vi "运行模式.vi"() -> (3 "单机运行":bool)   [LabVIEW 2014]
panel:
  in  "单机运行":bool
  in  "联机运行":bool
  # "请选择一种运行方式"
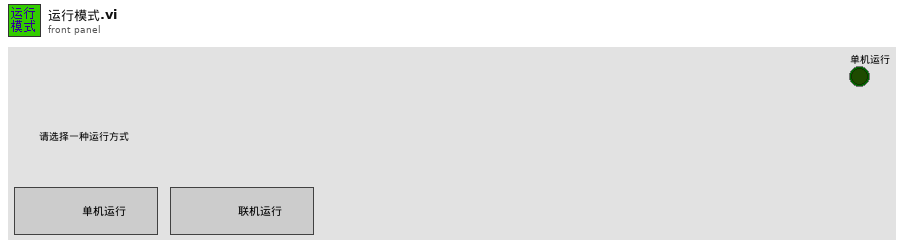
[diagram p1: front panel]
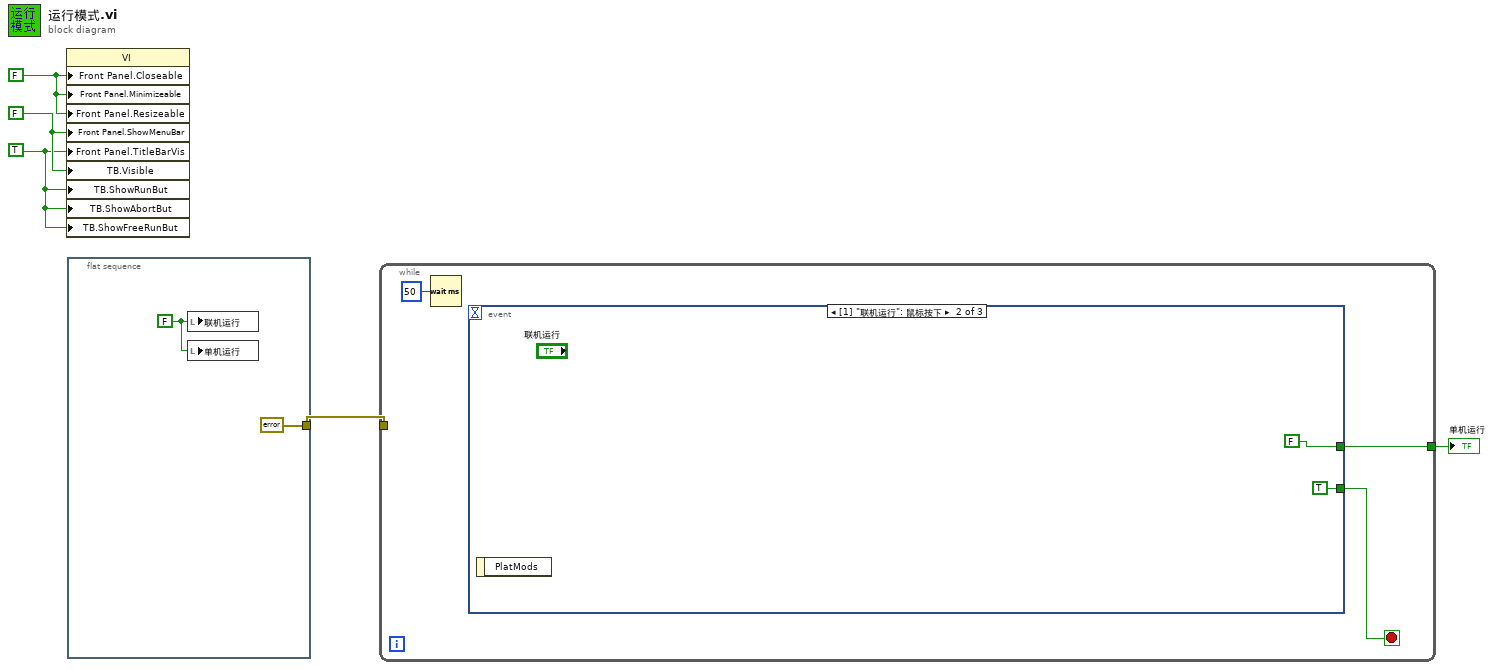
[diagram p0: block diagram]
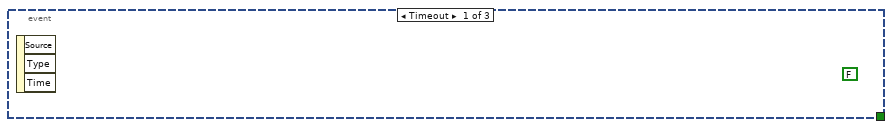
[diagram p2: hidden frame]
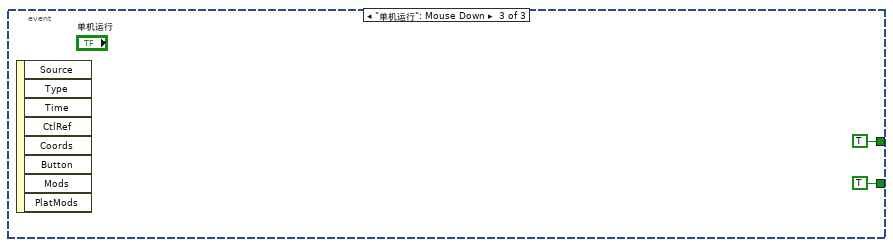
[diagram p3: hidden frame]
diagram:
  w3 = TRUE ("前面板窗口:可关闭")
  w2 = FALSE ("前面板窗口:可关闭")
  w4 = FALSE ("Front Panel Window:Closeable")
  n1 = property class="VI"("Front Panel.Closeable"=w2, "Front Panel.Minimizeable"=w2, "Front Panel.Resizeable"=w2, "Front Panel.ShowMenuBar"=w4, "Front Panel.TitleBarVis"=w3, "TB.Visible"=w4, "TB.ShowRunBut"=w3, "TB.ShowAbortBut"=w3, "TB.ShowFreeRunBut"=w3) -> ()  [unwired: 2 in, 2 out]
  n2 = flat-sequence {
    tunnel: [errorcluster {"status"=FALSE, "code"=0, "source"=""} ("错误常量")] -> w5
    frame #0 {
      w6 = FALSE ("扫码控制键")
      n3 = local write "联机运行"(w6) -> ()
      n4 = local write "单机运行"(w6) -> ()
    }
  }
  n5 = while {
    tunnel: w5 -> [_]
    tunnel: [w8] -> w1
    stop <- w9 stop-if-true
    n6 = Wait (ms)(milliseconds to wait=u32 50 ("等待时间（毫秒）")) -> ()  [unwired: 1 out]
    n7 = event shown="[1] \"联机运行\": 鼠标按下" {
      selector: _ -> [_ _ _]
      dyn-events: _ -> [_ _ _]
      timeout: _ -> [_ _ _]
      tunnel: [_ TRUE TRUE] -> w9
      tunnel: [_ FALSE TRUE] -> w8
      event Timeout {
        (unwired) FALSE
        n8 = event-data() -> ()  [unwired: 1 in, 3 out]
      }
      event "联机运行": Mouse Down {
        n9 = event-data() -> ()  [unwired: 1 in, 1 out]
      }
      event "单机运行": Mouse Down {
        n10 = event-data() -> ()  [unwired: 1 in, 8 out]
      }
    }
  }
  "单机运行" <- w1
